vi "Switching Levels Logic Test.vi"() -> ()   [LabVIEW 2018, in "Elevator.lvlib" / "Elevator.lvclass"]
uses:
  Elevator.lvclass
  Controls/Elevator Position.ctl
panel:
  in  "Hatch":bool
  out "Cargo/Hatch":T1
  in  "Up":bool
  in  "Down":bool
  in  "Toggle Cargo/Hatch":bool
  in  "stop":bool
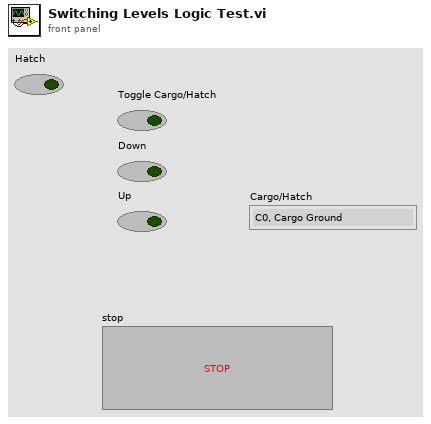
[diagram p1: front panel]
types:
  T1 = typedef "Elevator.lvlib/Elevator.lvclass/Elevator Position.ctl" = enum16{"C0, Cargo Ground", "C1, LV1 Cargo", "C2, Cargo Ship Cargo", "H0, LV1 Hatch", "H1, LV2 Hatch"}
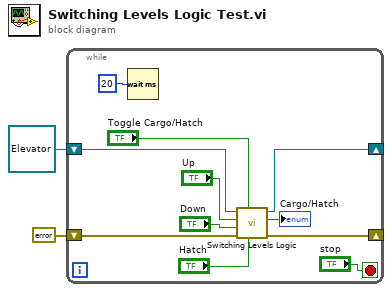
[diagram p0: block diagram]
diagram:
  n1 = while {
    shift-right: [w12] -> _
    shift-left: refnum<class "Elevator.lvclass"> refnum ("Elevator.lvlib:Elevator.lvclass") -> [w13]
    shift-right: [w9] -> _
    shift-left: errorcluster {"status"=FALSE, "code"=0, "source"=""} ("error in (no error)") -> [w10]
    stop <- "stop" stop-if-true
    n2 = Wait (ms)(milliseconds to wait=u32 20) -> ()  [unwired: 1 out]
    n3 = call "Switching Levels Logic.vi"("Hatch"="Hatch", "Cargo"="Toggle Cargo/Hatch", "error in (no error)"=w10, "Down"="Down", "Up"="Up", "Elevator in"=w13) -> ("error out"=w9:errorcluster, "Cargo/Hatch"=→"Cargo/Hatch":T1, "Elevator out"=w12:refnum<class "Elevator.lvclass">)  [unwired: 3 in]
  }
